vi "Auto 6.vi"(8 "Error In":errorcluster) -> (0 "Error Out":errorcluster)   [LabVIEW 2014]
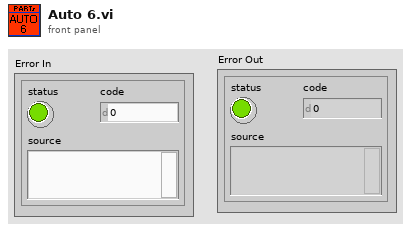
[diagram p1: front panel]
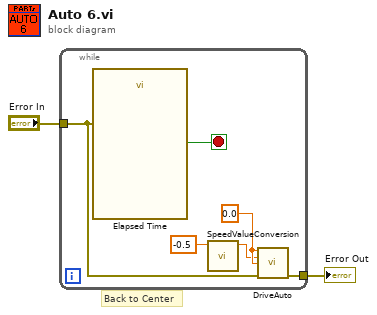
[diagram p0: block diagram]
diagram:
  # "Back to Center"
  n1 = while {
    tunnel: "Error In" -> [w5]
    tunnel: [w8] -> w2
    stop <- w6 stop-if-true
    w7 = 0.0 ("Arm Value")
    n2 = call "Elapsed Time"("error in (no error)"=w5) -> ("Time has Elapsed"=w6:bool)  [unwired: 11 in, 7 out]
    n3 = call "SpeedValueConversion.vi"("Motor Value In"=-0.5 ("X In")) -> ("New to Old Conversion Value Out"=w3:dbl)  [unwired: 9 in, 1 out]
    n4 = call "DriveAuto.vi"("X In"=w7, "Y In"=w3, "R In"=w7, "Error In"=w5) -> ("Error Out"=w8:errorcluster)  [unwired: 11 in]
  }
  "Error Out" <- w2
